vi "IsAttrMap.vi"(11 "Variant":variant) -> (2 "Map":T1, 3 "True":bool)   [LabVIEW 2019, in "lv-apt-json-file.lvlib"]
uses:
  lv-apt-json-file.lvlib
  Def-AttrMap -- Map.ctl
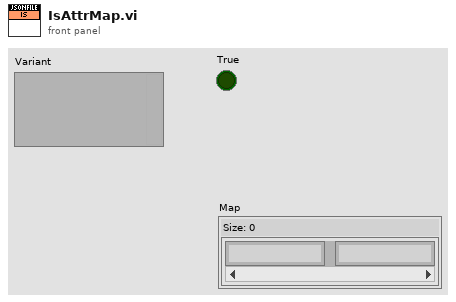
[diagram p1: front panel]
types:
  T1 = typedef "lv-apt-json-file.lvlib/Def-AttrMap -- Map.ctl" = map{string, string}
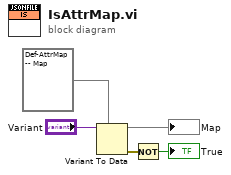
[diagram p0: block diagram]
diagram:
  n1 = Variant To Data(type=T1 {} ("Enum"), Variant="Variant") -> (data=→"Map":T1, error out=w3:errorcluster)  [unwired: 1 in]
  n2 = Not(x=w3) -> (.not. x?=→"True":bool)
